vi "AutoFollowAbsoluteTrajectory.vi"(6 "End Orientation":dbl, 7 "Orientation":T1, 8 "error in (no error)":errorcluster, 9 "TimeOut (s)":dbl, 11 "Trajectory":T2 {"States"."POSE"."ROTATION"."SIN" format="%13.4f"; "States"."POSE"."ROTATION"."COS" format="%13.4f"; "States"."POSE"."ROTATION"."VALUE" format="%13.4f"; "States"."POSE"."TRANSLATION"."Y" format="%14.3f"; "States"."POSE"."TRANSLATION"."X" format="%14.3f"; "TotalTImeSecs" format="%20.3f"}) -> (0 "error out":errorcluster)   [LabVIEW 2020]
doc: "Wrapper class for drive straight"
uses:
  <vilib>/Rock Robotics/WPI/ThirdParty/JAS_Junk/TrajLib/Trajectory_Library.lvlib
  <vilib>/Rock Robotics/WPI/ThirdParty/JAS_Junk/TrajLib/TypeDef/TRANSLATION2D.ctl
  <vilib>/Rock Robotics/WPI/ThirdParty/JAS_Junk/TrajLib/TypeDef/ROTATION2D.ctl
  <vilib>/Rock Robotics/WPI/ThirdParty/JAS_Junk/TrajLib/TypeDef/POSE2D.ctl
  <vilib>/Rock Robotics/WPI/ThirdParty/JAS_Junk/TrajLib/TypeDef/TRAJ_STATE.ctl
  <vilib>/Rock Robotics/WPI/ThirdParty/JAS_Junk/TrajLib/TypeDef/TRAJECTORY.ctl
  TrajectoryOrientation.ctl
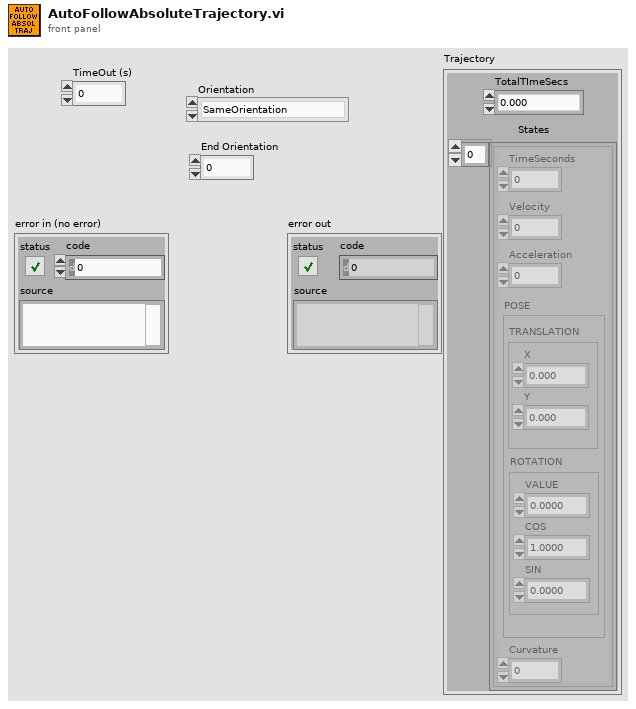
[diagram p1: front panel]
types:
  T1 = typedef "TrajectoryOrientation.ctl" = enum16{"SameOrientation", "RotateToEndOrientation"}
  T2 = typedef "Trajectory_Library.lvlib/TRAJECTORY.ctl" = cluster{"TotalTImeSecs":dbl, "States":T3[]}
  T3 = typedef "Trajectory_Library.lvlib/TRAJ_STATE.ctl" = cluster{"TimeSeconds":dbl, "Velocity":dbl, "Acceleration":dbl, "POSE":T4, "Curvature":dbl}
  T4 = typedef "Trajectory_Library.lvlib/POSE2D.ctl" = cluster{"TRANSLATION":T5, "ROTATION":T6}
  T5 = typedef "Trajectory_Library.lvlib/TRANSLATION2D.ctl" = cluster{"X":dbl, "Y":dbl}
  T6 = typedef "Trajectory_Library.lvlib/ROTATION2D.ctl" = cluster{"VALUE":dbl, "COS":dbl, "SIN":dbl}
  T7 = typedef "Trajectory_Library.lvlib/TIMER.ctl" = cluster{"StartTime":dbl, "Accumulated TIme":dbl, "Running":bool, "semaphore":T8}
  T8 = typedef "Semaphore RefNum" = refnum<k1>
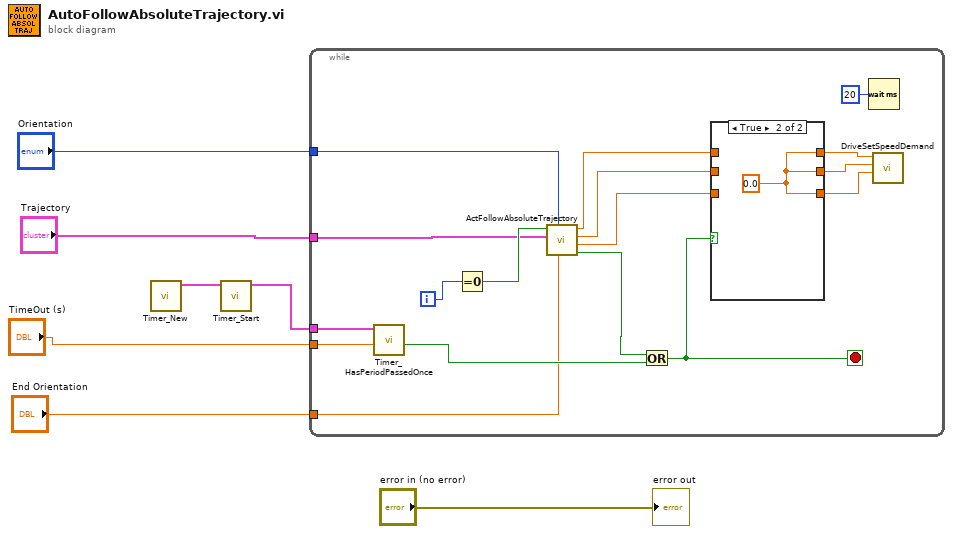
[diagram p0: block diagram]
diagram:
  n1 = call <vilib>:"Timer_New.vi"() -> ("TIMER"=w6:T7)  [unwired: 11 in]
  n2 = call <vilib>:"Timer_Start.vi"("in Timer"=w6) -> ("out Timer"=w5:T7)  [unwired: 10 in]
  n3 = while {
    tunnel: w5 -> [w23]
    tunnel: "TimeOut (s)" -> [w22]
    tunnel: "Trajectory" -> [w18]
    tunnel: "Orientation" -> [w9]
    tunnel: "End Orientation" -> [w8]
    i -> [w24]
    stop <- w10 stop-if-true
    n4 = call <vilib>:"Timer_HasPeriodPassedOnce.vi"("Period"=w22, "in Timer"=w23) -> ("Expired"=w21:bool)  [unwired: 7 in, 2 out]
    n5 = Equal To 0?(x=w24) -> (x = 0?=w19:bool)
    n6 = call "ActFollowAbsoluteTrajectory.vi"("End Orientation"=w8, "Orientation"=w9, "Trajectory"=w18, "FirstTime"=w19) -> ("Done"=w17:bool, "ASpeedDemand"=w16:dbl, "YSpeedDemand"=w15:dbl, "XSpeedDemand"=w14:dbl)  [unwired: 4 in]
    n7 = Or(x=w17, y=w21) -> (x .or. y?=w10:bool)
    n8 = case shown="True" w10 {
      tunnel: w14 -> [w27 _]
      tunnel: w15 -> [w26 _]
      tunnel: w16 -> [w25 _]
      tunnel: [w27 w28] -> w13
      tunnel: [w26 w28] -> w12
      tunnel: [w25 w28] -> w11
      frame False {
      }
      frame True {
        w28 = 0.0 ("XSpeedDemand")
      }
    }
    n9 = Wait (ms)(milliseconds to wait=u32 20) -> ()  [unwired: 1 out]
    n10 = call "DriveSetSpeedDemand.vi"("ASpeedDemand (d/s)"=w11, "YSpeedDemand (ft/s)"=w12, "XSpeedDemand (ft/s)"=w13) -> ()  [unwired: 9 in]
  }
  "error out" <- "error in (no error)"
